vi "Diode-Close.vi"(8 "error in (no error)":errorcluster, 11 "connection ID":refnum<k5>) -> (0 "error out":errorcluster)   [LabVIEW 2020]
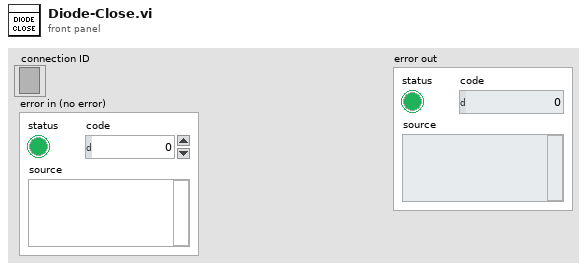
[diagram p1: front panel]
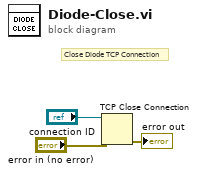
[diagram p0: block diagram]
diagram:
  # "Close Diode TCP Connection"
  n1 = TCP Close Connection(connection ID="connection ID", error in (no error)="error in (no error)") -> (error out=→"error out":errorcluster)  [unwired: 1 in, 1 out]
